vi "_FPGA_FinalCountdown.vi"(6 "Start":bool, 7 "Reset":bool, 10 "Countdown+1":u32=1) -> (1 "Idle":bool, 2 "Output":bool)   [LabVIEW 2018]
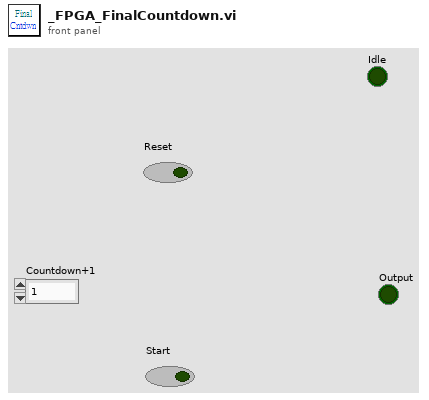
[diagram p1: front panel]
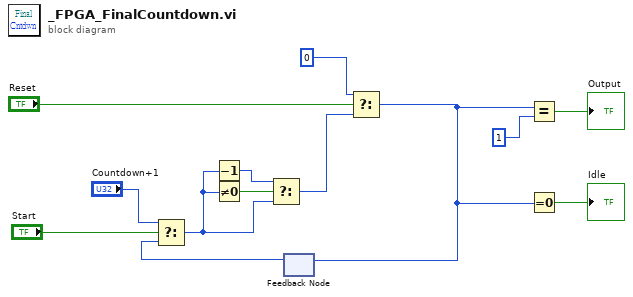
[diagram p0: block diagram]
diagram:
  n1 = feedback #1() -> (w11:u32)  [unwired: 1 in]
  n2 = Select(t="Countdown+1", s="Start", f=w11) -> (s? t:f=w6:u32)
  n3 = Decrement(x=w6) -> (x-1=w7:u32)
  n4 = Not Equal To 0?(x=w6) -> (x != 0?=w8:bool)
  n5 = Select(t=w7, s=w8, f=w6) -> (s? t:f=w5:u32)
  n6 = Select(t=u32 0, s="Reset", f=w5) -> (s? t:f=w2:u32)
  n7 = feedback-in #1(w2) -> ()
  n8 = Equal?(x=w2, y=u32 1) -> (x = y?=→"Output":bool)
  n9 = Equal To 0?(x=w2) -> (x = 0?=→"Idle":bool)
